vi "Notebook Find String.vi"(8 "error in (no error)":errorcluster, 11 ".NET Refnum in":refnum<k24>) -> (0 "error out":errorcluster, 1 "String location":i32, 2 "String to search for:":string, 3 ".NET Refnum out":refnum<k24>, 5 "Location after string":i32)   [LabVIEW 2021, in "Notebook.lvlib"]
uses:
  Notebook.lvlib
  System.Windows.Forms
  Strings/Strings.lvlib
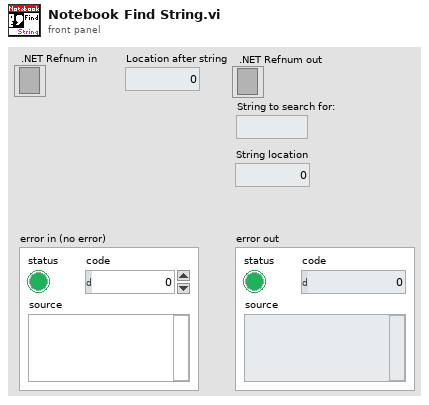
[diagram p1: front panel]
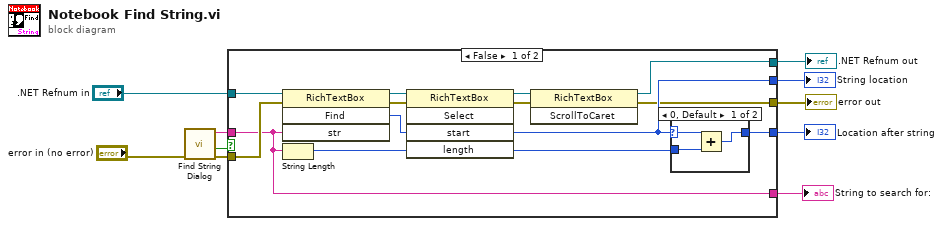
[diagram p0: block diagram]
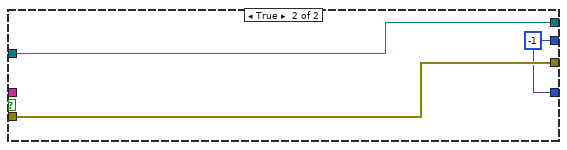
[diagram p3: hidden frame]
diagram:
  n1 = call "Find String Dialog.vi"("error in (no error)"="error in (no error)") -> ("error out"=w9:errorcluster, "Cancelled"=w2:bool, "String to search (out)"=w10:string)  [unwired: 8 in]
  n2 = case shown="False" w2 {
    tunnel: w10 -> [w11 _]
    tunnel: w9 -> [w19 w28]
    tunnel: ".NET Refnum in" -> [w18 w29]
    tunnel: [w17 w27] -> w6
    tunnel: [w16 w27] -> w5
    tunnel: [w13 w29] -> w4
    tunnel: [w12 w28] -> w3
    tunnel: [w11 _] -> w1
    frame False {
      n3 = invoke class="RichTextBox" method="Find"(reference=w18, error in=w19, "str"=w11) -> (reference out=w20:refnum<k24>, error out=w21:errorcluster, "Find"=w17:i32)  [unwired: 1 in, 1 out]
      n4 = String Length(string=w11) -> (length=w22:i32)
      n5 = invoke class="RichTextBox" method="Select"(reference=w20, error in=w21, "start"=w17, "length"=w22) -> (reference out=w15:refnum<k24>, error out=w14:errorcluster)  [unwired: 1 in, 3 out]
      n6 = invoke class="RichTextBox" method="ScrollToCaret"(reference=w15, error in=w14) -> (reference out=w13:refnum<k24>, error out=w12:errorcluster)  [unwired: 1 in, 1 out]
      n7 = case shown="0, Default" w17 {
        selector: w17 -> [w25 w26]
        tunnel: [w23 w26] -> w16
        tunnel: w22 -> [w24 _]
        frame 0, Default {
          n8 = Add(x=w25, y=w24) -> (x+y=w23:i32)
        }
        frame -1 {
        }
      }
    }
    frame True {
      w27 = -1 ("Find")
    }
  }
  "String to search for:" <- w1
  "String location" <- w6
  "error out" <- w3
  ".NET Refnum out" <- w4
  "Location after string" <- w5
